vi "aggregator - iii - real - atomic--TEST.vi"() -> ()   [LabVIEW 2014]
uses:
  interpolation state - real.ctl
  linear interpolation - real.vi
panel:
  out "state OUT":T1={"requested size"=20, "Array"=[], "actual number of elements"=0}
  in  "init?":bool
  out "interp average":dbl
  in  "number":dbl
  in  "requested size":i32=20
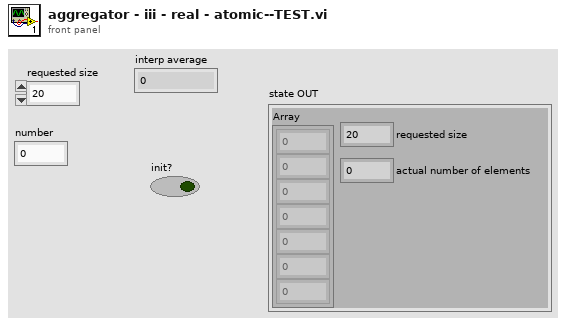
[diagram p1: front panel]
types:
  T1 = typedef "interpolation state - real.ctl" = cluster{"requested size":i32, "Array":dbl[], "actual number of elements":i32}
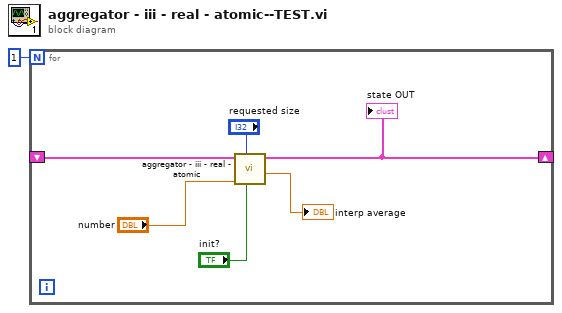
[diagram p0: block diagram]
diagram:
  n1 = for {
    N: 1 -> [_]
    shift-right: [w7] -> _
    shift-left: _ -> [w6]
    n2 = call "aggregator - iii - real - atomic.vi"("init?"="init?", "requested size"="requested size", "number IN"="number", "state IN"=w6) -> ("interp average"=→"interp average":dbl, "state OUT"=w7:T1)  [unwired: 3 in, 3 out]
    "state OUT" <- w7
  }
